vi "CAN Test.vi"(6 "Signal Write":dbl=77.0, 7 "Send Tx":bool, 9 "Tx Signal In":string="GIP_SetSerialNumber.vendorChar1", 11 "Interface":refnum<k21>="CAN1") -> (0 "error out":errorcluster)   [LabVIEW 2021, in "CAN wrapper.lvlib"]
uses:
  CAN wrapper.lvlib
  Private Controls/CAN States.ctl
  Private Controls/Setting.ctl
panel:
  out "Rx out Arr":dbl[](array[numeric])=[0.0, 81.0, 77.0, 0.0, 0.0]
  in  "Rx Array SN":string[](array[string])=["GIP_Status.GIP_State", "GIP_GetSerialNumber.vendorChar0", "GIP_GetSerialNumber.vendorChar1", "GIP_GetSerialNumber.vendorChar2", "GIP_GetSerialNumber.weekAndSerial"]
  in  "stop":bool
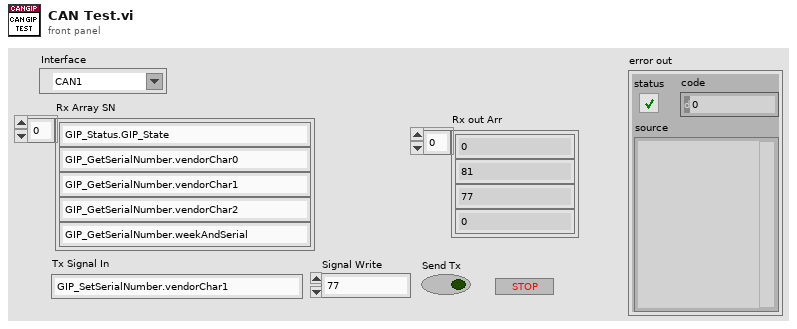
[diagram p1: front panel]
types:
  T1 = typedef "CAN wrapper.lvlib/CAN States.ctl" = enum16{"Init", "Rx Sess", "Tx Sess", "Read Signals", "Write Signals", "Close"}
  T2 = typedef "CAN wrapper.lvlib/Setting.ctl" = cluster{"Termination":u32, "Baud Rate":u64, "Interface":refnum<k21>, "XNET Database":refnum<k21>, "ECU":refnum<k21>}
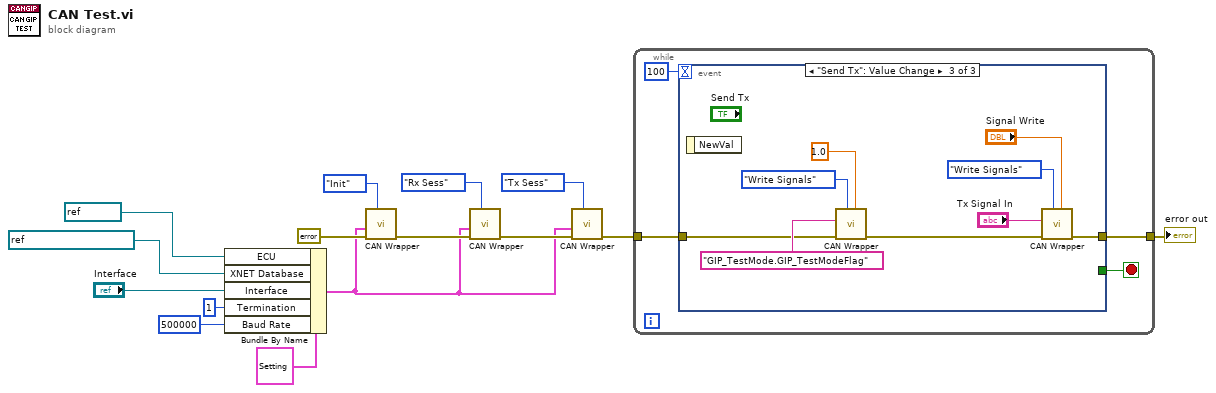
[diagram p0: block diagram]
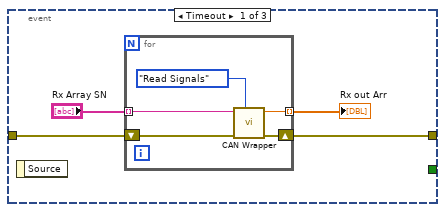
[diagram p2: hidden frame]
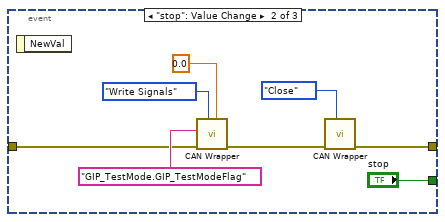
[diagram p3: hidden frame]
diagram:
  n1 = Bundle By Name(cluster=T2 {"Termination"=1, "Baud Rate"=125000, "Interface"="CAN1", "XNET Database"="GIP_CAN_Database", "ECU"="GIP\nGIP_CAN_Database"} ("Setting"), "ECU"=refnum<k21> "GIP\ncan_messages_818", "XNET Database"=refnum<k21> "can_messages_818", "Interface"="Interface", "Termination"=u32 1, "Baud Rate"=u64 500000) -> (w1:T2)
  n2 = call "CAN Wrapper.vi"("States"=CAN_States."Init" ("CAN States"), "error in"=errorcluster {"status"=FALSE, "code"=0, "source"=""}, "Setting"=w1) -> ("error out"=w14:errorcluster)  [unwired: 7 in, 1 out]
  n3 = call "CAN Wrapper.vi"("States"=CAN_States."Rx Sess" ("CAN States"), "error in"=w14, "Setting"=w1) -> ("error out"=w4:errorcluster)  [unwired: 7 in, 1 out]
  n4 = call "CAN Wrapper.vi"("States"=CAN_States."Tx Sess", "error in"=w4, "Setting"=w1) -> ("error out"=w3:errorcluster)  [unwired: 7 in, 1 out]
  n5 = while {
    tunnel: [w17] -> w6
    tunnel: w3 -> [w18]
    stop <- w19 stop-if-true
    n6 = event shown="[2] \"Send Tx\": Value Change" {
      selector: _ -> [_ _ _]
      dyn-events: _ -> [_ _ _]
      timeout: 100 -> [_ _ _]
      tunnel: [_ "stop" _] -> w19
      tunnel: w18 -> [w23 w31 w38]
      tunnel: [w22 w35 w43] -> w17
      event Timeout {
        n7 = event-data() -> ()  [unwired: 1 in, 1 out]
        n8 = for {
          tunnel: "Rx Array SN" -> [w26] mode=indexing
          tunnel: [w25] -> w21 mode=indexing
          shift-right: [w27] -> w22
          shift-left: w23 -> [w28]
          n9 = call "CAN Wrapper.vi"("States"=CAN_States."Read Signals" ("CAN States"), "error in"=w28, "Rx Signal In"=w26) -> ("error out"=w27:errorcluster, "Signal out"=w25:dbl)  [unwired: 7 in]
        }
        "Rx out Arr" <- w21
      }
      event "stop": Value Change {
        n10 = event-data() -> ()  [unwired: 1 in, 1 out]
        n11 = call "CAN Wrapper.vi"("Signal Write"=0.0, "States"=CAN_States."Write Signals" ("CAN States"), "error in"=w31, "Tx Signal In"="GIP_TestMode.GIP_TestModeFlag") -> ("error out"=w30:errorcluster)  [unwired: 6 in, 1 out]
        n12 = call "CAN Wrapper.vi"("States"=CAN_States."Close" ("CAN States"), "error in"=w30) -> ("error out"=w35:errorcluster)  [unwired: 8 in, 1 out]
      }
      event "Send Tx": Value Change {
        n13 = event-data() -> ()  [unwired: 1 in, 1 out]
        n14 = call "CAN Wrapper.vi"("Signal Write"=1.0, "States"=CAN_States."Write Signals" ("CAN States"), "error in"=w38, "Tx Signal In"="GIP_TestMode.GIP_TestModeFlag") -> ("error out"=w37:errorcluster)  [unwired: 6 in, 1 out]
        n15 = call "CAN Wrapper.vi"("Signal Write"="Signal Write", "States"=CAN_States."Write Signals" ("CAN States"), "error in"=w37, "Tx Signal In"="Tx Signal In") -> ("error out"=w43:errorcluster)  [unwired: 6 in, 1 out]
      }
    }
  }
  "error out" <- w6
